vi "ConvertToR2DeviceModel.vi"(11 "DeviceModel":T1) -> (3 "R2 DeviceModel":T14)   [LabVIEW 2017, in "ServerComm.lvlib"]
uses:
  <vilib>/addons/InsightCM/Devices/Shared/Common/ServerComm/ServerComm.lvlib
  <vilib>/addons/InsightCM/MessageBus/Base/controls/R2_DeviceModel.ctl
  <vilib>/addons/InsightCM/MessageBus/Base/controls/R2_Device.ctl
  <vilib>/addons/InsightCM/MessageBus/Base/controls/KeyValuePair.ctl
  <vilib>/addons/InsightCM/MessageBus/Base/controls/DeviceState.ctl
  <vilib>/addons/InsightCM/MessageBus/Base/controls/R2_DataGroup.ctl
  <vilib>/addons/InsightCM/MessageBus/Base/controls/OperatingState.ctl
  <vilib>/addons/InsightCM/MessageBus/Base/controls/Trigger.ctl
  <vilib>/addons/InsightCM/MessageBus/Base/controls/Condition.ctl
  <vilib>/addons/InsightCM/MessageBus/Base/controls/BurstModeTrigger.ctl
  <vilib>/addons/InsightCM/MessageBus/Base/controls/DeviceSensorGroup.ctl
  <vilib>/addons/InsightCM/MessageBus/Base/controls/WirelessEndpoint.ctl
  <vilib>/addons/InsightCM/MessageBus/Base/controls/WirelessChannel.ctl
  <vilib>/addons/InsightCM/MessageBus/Base/controls/R2_Channel.ctl
  <vilib>/addons/InsightCM/MessageBus/Base/controls/Metric.ctl
  <vilib>/addons/InsightCM/MessageBus/Base/controls/Tag.ctl
  <vilib>/addons/InsightCM/MessageBus/Base/controls/DeviceModel.ctl
  <vilib>/addons/InsightCM/MessageBus/Base/controls/Device.ctl
  <vilib>/addons/InsightCM/MessageBus/Base/controls/DataGroup.ctl
  <vilib>/addons/InsightCM/MessageBus/Base/controls/Channel.ctl
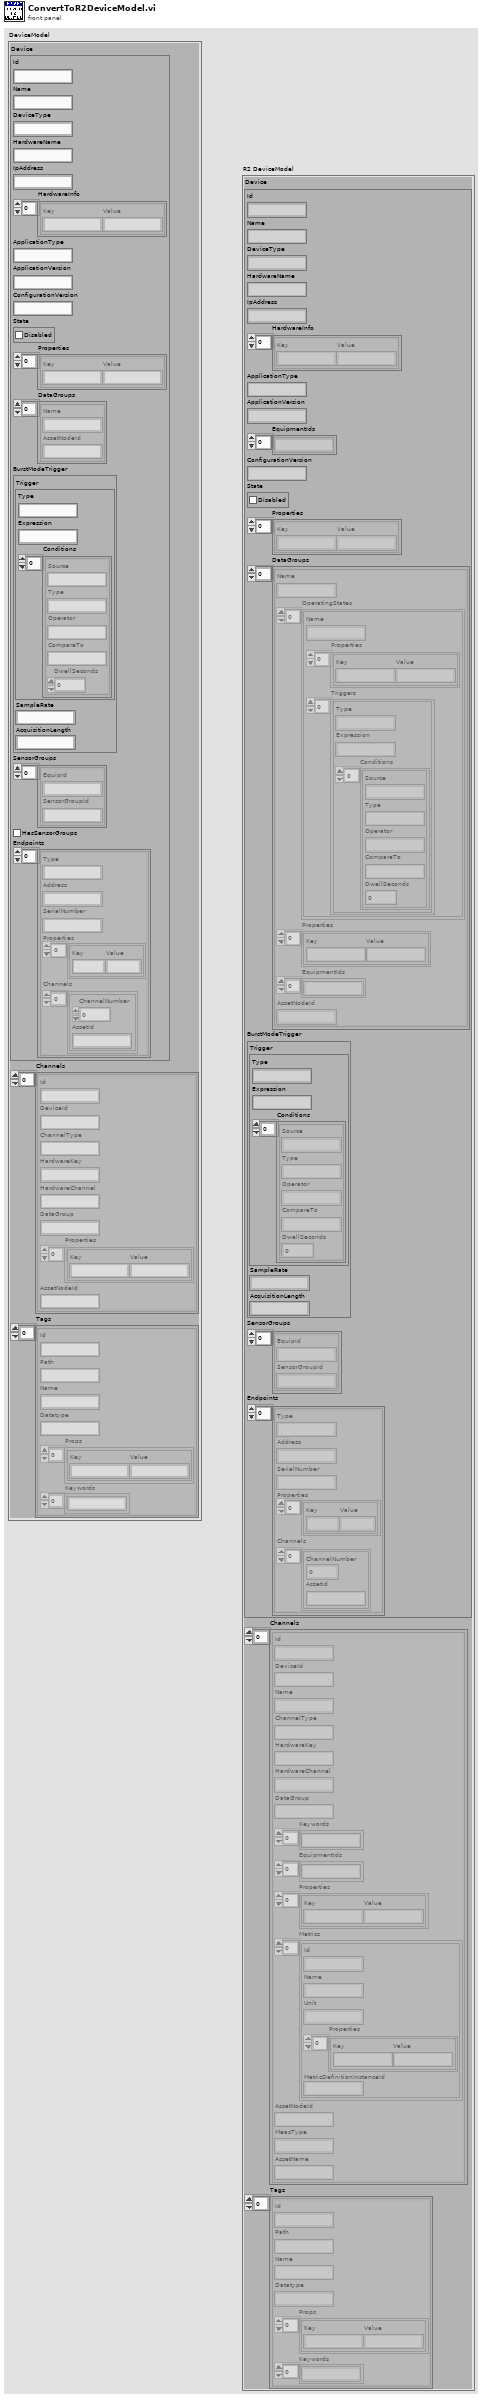
[diagram p1: front panel]
types:
  T1 = typedef "DeviceModel.ctl" = cluster{"Device":T2, "Channels":T12[], "Tags":T13[]}
  T2 = typedef "Device.ctl" = cluster{"Id":string, "Name":string, "DeviceType":string, "HardwareName":string, "IpAddress":string, "HardwareInfo":T3[], "ApplicationType":string, "ApplicationVersion":string, "ConfigurationVersion":string, "State":T4, "Properties":T3[], "DataGroups":T5[], "BurstModeTrigger":T6, "SensorGroups":T9[], "HasSensorGroups":bool, "Endpoints":T10[]}
  T3 = typedef "KeyValuePair.ctl" = cluster{"Key":string, "Value":string}
  T4 = typedef "DeviceState.ctl" = cluster{"Disabled":bool}
  T5 = typedef "DataGroup.ctl" = cluster{"Name":string, "AssetNodeId":string}
  T6 = typedef "BurstModeTrigger.ctl" = cluster{"Trigger":T7, "SampleRate":string, "AcquisitionLength":string}
  T7 = typedef "Trigger.ctl" = cluster{"Type":string, "Expression":string, "Conditions":T8[]}
  T8 = typedef "Condition.ctl" = cluster{"Source":string, "Type":string, "Operator":string, "CompareTo":string, "DwellSeconds":dbl}
  T9 = typedef "DeviceSensorGroup.ctl" = cluster{"EquipId":string, "SensorGroupId":string}
  T10 = typedef "WirelessEndpoint.ctl" = cluster{"Type":string, "Address":string, "SerialNumber":string, "Properties":T3[], "Channels":T11[]}
  T11 = typedef "WirelessChannel.ctl" = cluster{"ChannelNumber":i32, "AssetId":string}
  T12 = typedef "Channel.ctl" = cluster{"Id":string, "DeviceId":string, "ChannelType":string, "HardwareKey":string, "HardwareChannel":string, "DataGroup":string, "Properties":T3[], "AssetNodeId":string}
  T13 = typedef "Tag.ctl" = cluster{"Id":string, "Path":string, "Name":string, "Datatype":string, "Props":T3[], "Keywords":string[]}
  T14 = typedef "R2_DeviceModel.ctl" = cluster{"Device":T15, "Channels":T18[], "Tags":T13[]}
  T15 = typedef "R2_Device.ctl" = cluster{"Id":string, "Name":string, "DeviceType":string, "HardwareName":string, "IpAddress":string, "HardwareInfo":T3[], "ApplicationType":string, "ApplicationVersion":string, "EquipmentIds":string[], "ConfigurationVersion":string, "State":T4, "Properties":T3[], "DataGroups":T16[], "BurstModeTrigger":T6, "SensorGroups":T9[], "Endpoints":T10[]}
  T16 = typedef "R2_DataGroup.ctl" = cluster{"Name":string, "OperatingStates":T17[], "Properties":T3[], "EquipmentIds":string[], "AssetNodeId":string}
  T17 = typedef "OperatingState.ctl" = cluster{"Name":string, "Properties":T3[], "Triggers":T7[]}
  T18 = typedef "R2_Channel.ctl" = cluster{"Id":string, "DeviceId":string, "Name":string, "ChannelType":string, "HardwareKey":string, "HardwareChannel":string, "DataGroup":string, "Keywords":string[], "EquipmentIds":string[], "Properties":T3[], "Metrics":T19[], "AssetNodeId":string, "MeasType":string, "AssetName":string}
  T19 = typedef "Metric.ctl" = cluster{"Id":string, "Name":string, "Unit":string, "Properties":T3[], "MetricDefinitionInstanceId":string}
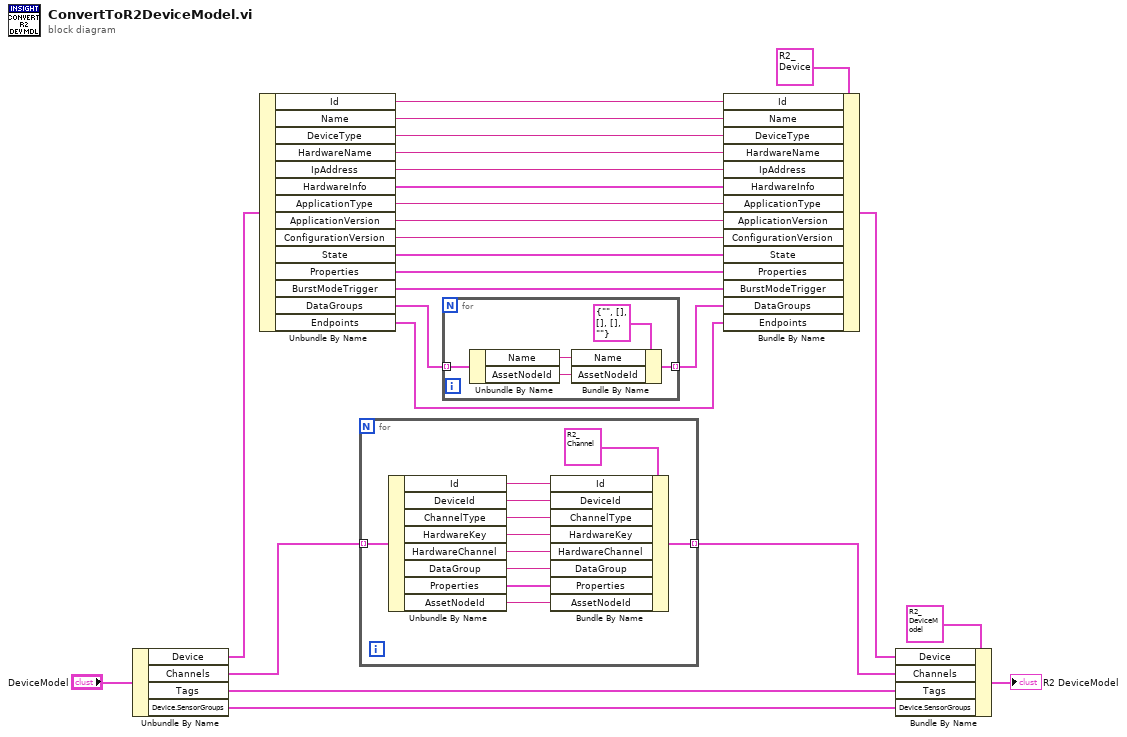
[diagram p0: block diagram]
diagram:
  n1 = Unbundle By Name("DeviceModel") -> ("Device"=w20:T2, "Channels"=w7:T12[], "Tags"=w8:T13[], "Device.SensorGroups"=w2:T9[])
  n2 = Unbundle By Name(w20) -> ("Id"=w9:string, "Name"=w10:string, "DeviceType"=w11:string, "HardwareName"=w12:string, "IpAddress"=w13:string, "HardwareInfo"=w14:T3[], "ApplicationType"=w15:string, "ApplicationVersion"=w16:string, "ConfigurationVersion"=w17:string, "State"=w18:T4, "Properties"=w19:T3[], "BurstModeTrigger"=w3:T6, "DataGroups"=w4:T5[], "Endpoints"=w1:T10[])
  n3 = for {
    tunnel: [w35] -> w21 mode=indexing
    tunnel: w7 -> [w34] mode=indexing
    n4 = Unbundle By Name(w34) -> ("Id"=w33:string, "DeviceId"=w32:string, "ChannelType"=w31:string, "HardwareKey"=w30:string, "HardwareChannel"=w29:string, "DataGroup"=w28:string, "Properties"=w27:T3[], "AssetNodeId"=w26:string)
    n5 = Bundle By Name(cluster=T18 {"Id"="", "DeviceId"="", "Name"="", "ChannelType"="", "HardwareKey"="", "HardwareChannel"="", "DataGroup"="", "Keywords"=[], "EquipmentIds"=[], "Properties"=[], "Metrics"=[], "AssetNodeId"="", "MeasType"="", "AssetName"=""} ("ChannelModel"), "Id"=w33, "DeviceId"=w32, "ChannelType"=w31, "HardwareKey"=w30, "HardwareChannel"=w29, "DataGroup"=w28, "Properties"=w27, "AssetNodeId"=w26) -> (w35:T18)
  }
  n6 = for {
    tunnel: w4 -> [w40] mode=indexing
    tunnel: [w37] -> w5 mode=indexing
    n7 = Unbundle By Name(w40) -> ("Name"=w39:string, "AssetNodeId"=w38:string)
    n8 = Bundle By Name(cluster=T16 {"Name"="", "OperatingStates"=[], "Properties"=[], "EquipmentIds"=[], "AssetNodeId"=""} ("DataGroup"), "Name"=w39, "AssetNodeId"=w38) -> (w37:T16)
  }
  n9 = Bundle By Name(cluster=T15 {"Id"="", "Name"="", "DeviceType"="", "HardwareName"="", "IpAddress"="", "HardwareInfo"=[], "ApplicationType"="", "ApplicationVersion"="", "EquipmentIds"=[], "ConfigurationVersion"="", "State"={"Disabled"=FALSE}, "Properties"=[], "DataGroups"=[], "BurstModeTrigger"={"Trigger"={"Type"="", "Expression"="", "Conditions"=[]}, "SampleRate"="", "AcquisitionLength"=""}, "SensorGroups"=[], "Endpoints"=[]} ("Device"), "Id"=w9, "Name"=w10, "DeviceType"=w11, "HardwareName"=w12, "IpAddress"=w13, "HardwareInfo"=w14, "ApplicationType"=w15, "ApplicationVersion"=w16, "ConfigurationVersion"=w17, "State"=w18, "Properties"=w19, "BurstModeTrigger"=w3, "DataGroups"=w5, "Endpoints"=w1) -> (w22:T15)
  n10 = Bundle By Name(cluster=T14 {"Device"={"Id"="", "Name"="", "DeviceType"="", "HardwareName"="", "IpAddress"="", "HardwareInfo"=[], "ApplicationType"="", "ApplicationVersion"="", "EquipmentIds"=[], "ConfigurationVersion"="", "State"={"Disabled"=FALSE}, "Properties"=[], "DataGroups"=[], "BurstModeTrigger"={"Trigger"={"Type"="", "Expression"="", "Conditions"=[]}, "SampleRate"="", "AcquisitionLength"=""}, "SensorGroups"=[], "Endpoints"=[]}, "Channels"=[], "Tags"=[]} ("R2 DeviceModel"), "Device"=w22, "Channels"=w21, "Tags"=w8, "Device.SensorGroups"=w2) -> (→"R2 DeviceModel":T14)
